vi "time_adding_loop.vi"(10 "times":string[](array[string])) -> (2 "Total time":dbl)   [LabVIEW 2015]
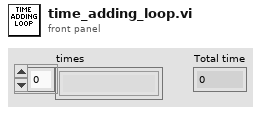
[diagram p1: front panel]
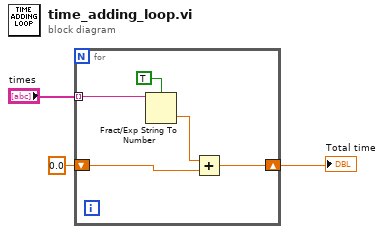
[diagram p0: block diagram]
diagram:
  n1 = for {
    tunnel: "times" -> [w8] mode=indexing
    shift-right: [w5] -> w3
    shift-left: 0.0 -> [w4]
    n2 = Fract/Exp String To Number(use system decimal point (T)=TRUE, string=w8) -> (number=w6:dbl)  [unwired: 2 in, 1 out]
    n3 = Add(x=w6, y=w4) -> (x+y=w5:dbl)
  }
  "Total time" <- w3
